vi "BBoxLiteLabViewTest.vi"() -> ()   [LabVIEW 2019]
uses:
  Y:/Codebase/bbox-api/example/LabView2019_BBoxLite/BBoxAPI.dll
  BBoxAPI.dll
panel:
  in  "SN2( Input by user)":string
  out "SN2 ret value":string
  in  "SN2 Ang ( Input by user) 2":dbl
  in  "SN2 dB( Input by user)":dbl
  in  "SN1( Input by user)":string
  out "Init Info":string
  out "SN1 ret value":string
  in  "SN1 Ang ( Input by user)":dbl
  in  "SN1 dB( Input by user)":dbl
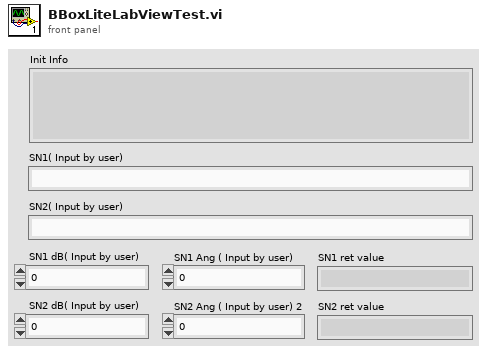
[diagram p1: front panel]
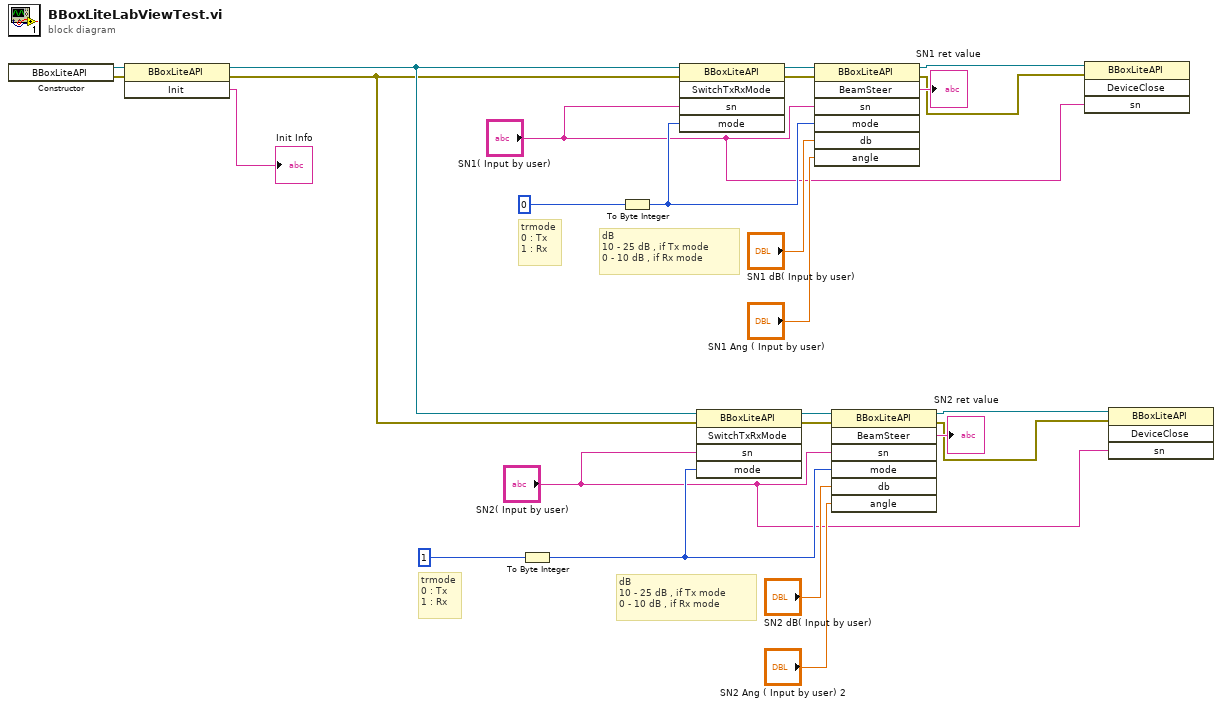
[diagram p0: block diagram]
diagram:
  # "dB\n10 - 25 dB , if Tx mode\n0 - 10 dB , if Rx mode"
  # "trmode\n0 : Tx\n1 : Rx"
  # "dB\n10 - 25 dB , if Tx mode\n0 - 10 dB , if Rx mode"
  # "trmode\n0 : Tx\n1 : Rx"
  n1 = constructor class="BBoxLiteAPI"() -> (reference out=w22:refnum<k24>, error out=w21:errorcluster)  [unwired: 3 in, 1 out]
  n2 = invoke class="BBoxLiteAPI" method="Init"(reference=w22, error in=w21) -> (reference out=w8:refnum<k24>, error out=w7:errorcluster, "Init"=→"Init Info":string)  [unwired: 1 in]
  n3 = To Byte Integer(number=1) -> (8bit integer=w11:i8)
  n4 = To Byte Integer(number=0) -> (8bit integer=w18:i8)
  n5 = invoke class="BBoxLiteAPI" method="SwitchTxRxMode"(reference=w8, error in=w7, "sn"="SN1( Input by user)", "mode"=w18) -> (reference out=w24:refnum<k24>, error out=w23:errorcluster)  [unwired: 1 in, 3 out]
  n6 = invoke class="BBoxLiteAPI" method="SwitchTxRxMode"(reference=w8, error in=w7, "sn"="SN2( Input by user)", "mode"=w11) -> (reference out=w14:refnum<k24>, error out=w13:errorcluster)  [unwired: 1 in, 3 out]
  n7 = invoke class="BBoxLiteAPI" method="BeamSteer"(reference=w24, error in=w23, "sn"="SN1( Input by user)", "mode"=w18, "db"="SN1 dB( Input by user)", "angle"="SN1 Ang ( Input by user)") -> (reference out=w6:refnum<k24>, error out=w5:errorcluster, "BeamSteer"=→"SN1 ret value":string)  [unwired: 1 in, 4 out]
  n8 = invoke class="BBoxLiteAPI" method="BeamSteer"(reference=w14, error in=w13, "sn"="SN2( Input by user)", "mode"=w11, "db"="SN2 dB( Input by user)", "angle"="SN2 Ang ( Input by user) 2") -> (reference out=w3:refnum<k24>, error out=w2:errorcluster, "BeamSteer"=→"SN2 ret value":string)  [unwired: 1 in, 4 out]
  n9 = invoke class="BBoxLiteAPI" method="DeviceClose"(reference=w6, error in=w5, "sn"="SN1( Input by user)") -> ()  [unwired: 1 in, 4 out]
  n10 = invoke class="BBoxLiteAPI" method="DeviceClose"(reference=w3, error in=w2, "sn"="SN2( Input by user)") -> ()  [unwired: 1 in, 4 out]
